vi "GenerateDefaultChannelList.vi"() -> (3 "default channel list":string[](array[string]))   [LabVIEW 2017, in "McsaFpgaAcquisition.lvlib"]
uses:
  <vilib>/addons/InsightCM/Devices/Shared/Mcsa/McsaFpgaAcquisition/McsaFpgaAcquisition.lvlib
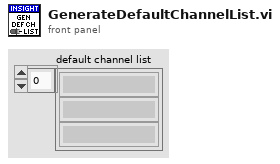
[diagram p1: front panel]
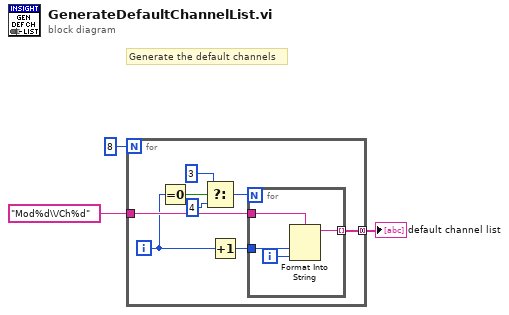
[diagram p0: block diagram]
diagram:
  # "Generate the default channels"
  n1 = for {
    N: 8 -> [_]
    tunnel: "Mod%d\\/Ch%d" -> [w11]
    tunnel: [w9] -> w1 mode=concatenating
    i -> [w4]
    n2 = Equal To 0?(x=w4) -> (x = 0?=w5:bool)
    n3 = Select(t=3, s=w5, f=4) -> (s? t:f=w7:i32)
    n4 = Increment(x=w4) -> (x+1=w10:i32)
    n5 = for {
      N: w7 -> [_]
      tunnel: w11 -> [w15]
      tunnel: w10 -> [w13]
      tunnel: [w12] -> w9 mode=indexing
      i -> [w14]
      n6 = Format Into String(format string=w15, w13, w14) -> (resulting string=w12:string)  [unwired: 2 in, 1 out]
    }
  }
  "default channel list" <- w1
